vi "IncrementQueue.vi"(9 "is sequence running ?":bool=TRUE, 10 "acquisition frame":T1, 11 "queue in":refnum<queue>) -> (3 "queue out":refnum<queue>)   [LabVIEW 2018]
uses:
  typedef/AcquisitionFrame.ctl
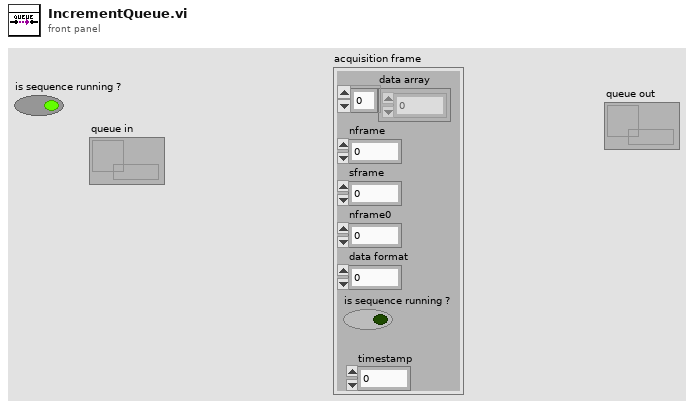
[diagram p1: front panel]
types:
  T1 = typedef "AcquisitionFrame.ctl" = cluster{"data array":u8[], "nframe":i32, "sframe":i32, "nframe0":i32, "data format":i32, "is sequence running ?":bool, "timestamp":dbl}
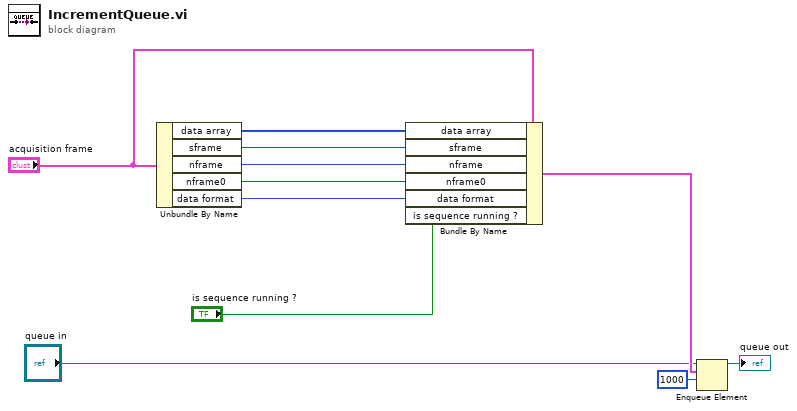
[diagram p0: block diagram]
diagram:
  n1 = Unbundle By Name("acquisition frame") -> ("data array"=w9:u8[], "sframe"=w8:i32, "nframe"=w7:i32, "nframe0"=w6:i32, "data format"=w5:i32)
  n2 = Bundle By Name(cluster="acquisition frame", "data array"=w9, "sframe"=w8, "nframe"=w7, "nframe0"=w6, "data format"=w5, "is sequence running ?"="is sequence running ?") -> (w3:T1)
  n3 = Enqueue Element(queue="queue in", element=w3, timeout in ms (-1)=1000) -> (queue out=→"queue out":refnum<queue>)  [unwired: 1 in, 2 out]
